vi "Point Shoot Markers.vi"(8 "Error in (no error)":errorcluster, 9 "Y":dbl=3.1847341119828343e-07, 10 "X":dbl=-2.397470098003396e-07, 11 "Method":enum16{"init", "run", "end"}(ring)=enum."run") -> (0 "Error out":errorcluster)   [LabVIEW 2014]
doc: "Example of a measurement VI to be used in the \"Point & Shoot\" tool in Follow Me mode as external VI.\n\nThis example performs multiple bias spectroscopy measurements after each movement.\n\n- Nanonis Programming Interface -"
uses:
  <userlib>/Nanonis Prog Interface V5/Nanonis Prog Interface.lvlib
panel:
  in  "NumPoints":i32=2
  in  "startText":string="start"
  in  "Color":u32(colorbox)=14680303
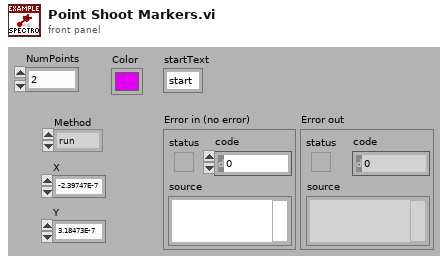
[diagram p1: front panel]
types:
  T1 = cluster{"X (m)":sgl, "Y (m)":sgl, "Text":string, "Color":u32, "Visible":bool}[]
  T2 = cluster{"X (m)":sgl, "Y (m)":sgl, "Text":string, "Color":u32, "Visible":bool}
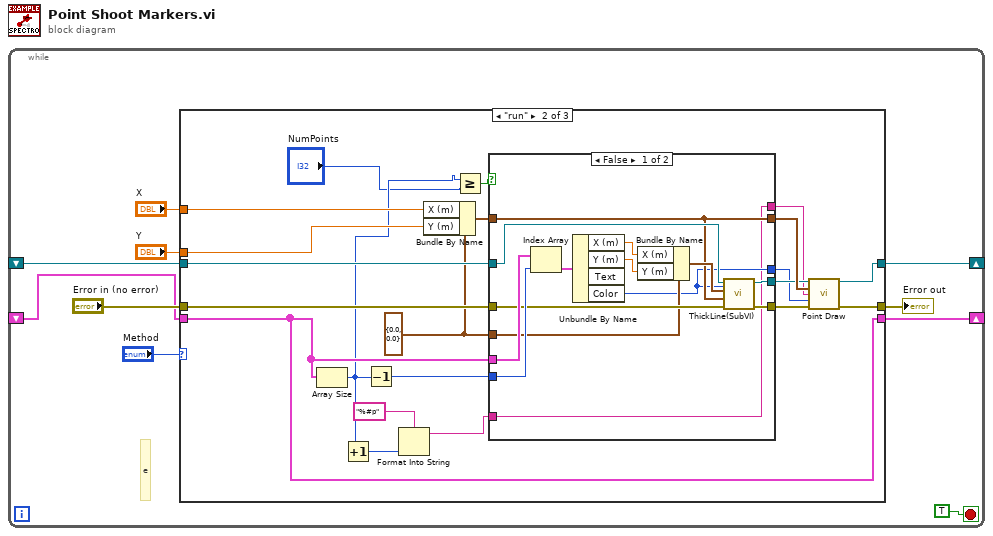
[diagram p0: block diagram]
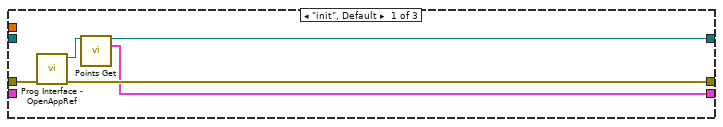
[diagram p2: hidden frame]
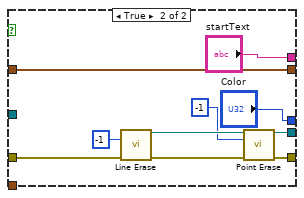
[diagram p3: hidden frame]
diagram:
  n1 = while {
    shift-right: [w4] -> _
    shift-left: _ -> [w3]
    shift-right: [w2] -> _
    shift-left: _ -> [w1]
    stop <- TRUE stop-if-true
    # "e"
    n2 = case shown="\"run\"" "Method" {
      tunnel: "Error in (no error)" -> [w15 w34 w63]
      tunnel: [w14 w33 w63] -> w7
      tunnel: "X" -> [_ w30 _]
      tunnel: "Y" -> [_ w31 _]
      tunnel: [w12 w36 w62] -> w4
      tunnel: w3 -> [_ w35 w62]
      tunnel: [w11 w32 w61] -> w2
      tunnel: w1 -> [_ w32 w61]
      frame "init", Default {
        n3 = call <userlib>:"Prog Interface - OpenAppRef.vi"("Error in (no error)"=w15) -> ("Error out"=w14:errorcluster, "Application reference"=w13:refnum<vi>)  [unwired: 5 in]
        n4 = call <userlib>:"Points Get.vi"("Application ref in"=w13) -> ("Application ref out"=w12:refnum<vi>, "Points"=w11:T1)  [unwired: 12 in, 1 out]
      }
      frame "run" {
        w24 = cluster{"X (m)":sgl, "Y (m)":sgl} {"X (m)"=0.0, "Y (m)"=0.0} ("End Point Coordinates")
        n5 = Array Size(array=w32) -> (size(s)=w19:i32)
        n6 = Increment(x=w19) -> (x+1=w16:i32)
        n7 = Decrement(x=w19) -> (x-1=w29:i32)
        n8 = Format Into String(format string="%#p", w16) -> (resulting string=w22:string)  [unwired: 2 in, 1 out]
        n9 = Bundle By Name(cluster=w24, "X (m)"=w30, "Y (m)"=w31) -> (w23:cluster{"X (m)":sgl, "Y (m)":sgl})
        n10 = Greater Or Equal?(x=w19, y="NumPoints") -> (x >= y?=w17:bool)
        n11 = case shown="False" w17 {
          tunnel: w32 -> [w50 _]
          tunnel: w29 -> [w49 _]
          tunnel: [w39 w54] -> w28
          tunnel: w35 -> [w44 _]
          tunnel: [w43 w56] -> w27
          tunnel: w34 -> [w42 w55]
          tunnel: [w41 w51] -> w26
          tunnel: w24 -> [w40 _]
          tunnel: w23 -> [w39 w54]
          tunnel: w22 -> [w37 _]
          tunnel: [w37 "startText"] -> w21
          tunnel: [w38 "Color"] -> w20
          frame False {
            n12 = Index Array(array=w50, index=w49) -> (element=w48:T2)
            n13 = Unbundle By Name(w48) -> ("X (m)"=w47:sgl, "Y (m)"=w46:sgl, "Color"=w38:u32)  [unwired: 1 out]
            n14 = Bundle By Name(cluster=w40, "X (m)"=w47, "Y (m)"=w46) -> (w45:cluster{"X (m)":sgl, "Y (m)":sgl})
            n15 = call "ThickLine(SubVI).vi"("Color"=w38, "error in (no error)"=w42, "End Point Coordinates"=w39, "End Point Coordinates 2"=w45, "Application in"=w44) -> ("error out"=w41:errorcluster, "Application out"=w43:refnum<vi>)  [unwired: 5 in]
          }
          frame True {
            n16 = call <userlib>:"Line Erase.vi"("Line index (-1=All lines)"=-1, "error in (no error)"=w55) -> ("Application ref out"=w60:refnum<vi>, "error out"=w59:errorcluster)  [unwired: 12 in]
            n17 = call <userlib>:"Point Erase.vi"("Application ref in"=w60, "Point index (-1=All points)"=-1, "error in (no error)"=w59) -> ("Application ref out"=w56:refnum<vi>, "error out"=w51:errorcluster)  [unwired: 11 in]
          }
        }
        n18 = call <userlib>:"Point Draw.vi"("Application ref in"=w27, "Point Coordinates"=w28, "Text"=w21, "Color"=w20, "error in (no error)"=w26) -> ("Application ref out"=w36:refnum<vi>, "error out"=w33:errorcluster)  [unwired: 9 in]
      }
      frame "end" {
      }
    }
    "Error out" <- w7
  }
